vi "GSTOP RESET.vi"(1 "index(-1 for All)":i32=-1, 7 "error in (no error)":errorcluster) -> (8 "error out":errorcluster)   [LabVIEW 2017, in "GSTOP.lvlib"]
doc: "Resets a stop flag to FALSE; Index=-1 means reset the global stop flag.\n------\n将停止位复位为 FALSE；Index=-1 表示复位全局停止位。"
uses:
  GSTOP.lvlib
  _def_oper.ctl
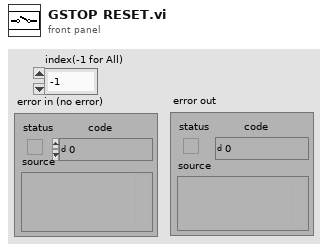
[diagram p1: front panel]
types:
  T1 = typedef "GSTOP.lvlib/_def_oper.ctl" = enum16{"init", "reset", "get", "set"}
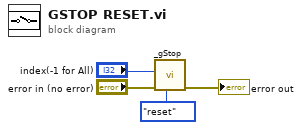
[diagram p0: block diagram]
diagram:
  n1 = call "_gStop.vi"("op"=_def_oper."reset", "error in (no error)"="error in (no error)", "index(-1 for All)"="index(-1 for All)") -> ("error out"=→"error out":errorcluster)  [unwired: 7 in, 1 out]
